vi "Select_Desired_Indicies.vi"(5 "No of averages":i32=1, 7 "Clients time":dbl, 8 "End time":dbl, 9 "Start time":dbl, 10 "Table values":dbl[][](array[numeric]) format="%.2f") -> (0 "Length":i32[](array[numeric]), 1 "End Integer":i32[](array[numeric]), 2 "Start integer":i32[](array[numeric]), 3 "Averaging Times":dbl[](array[numeric]) format="%.2f", 4 "Client leads me by:":dbl, 6 "Total Time":dbl format="%.2f")   [LabVIEW 2021]
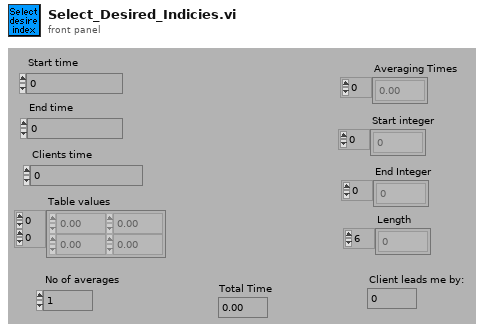
[diagram p1: front panel]
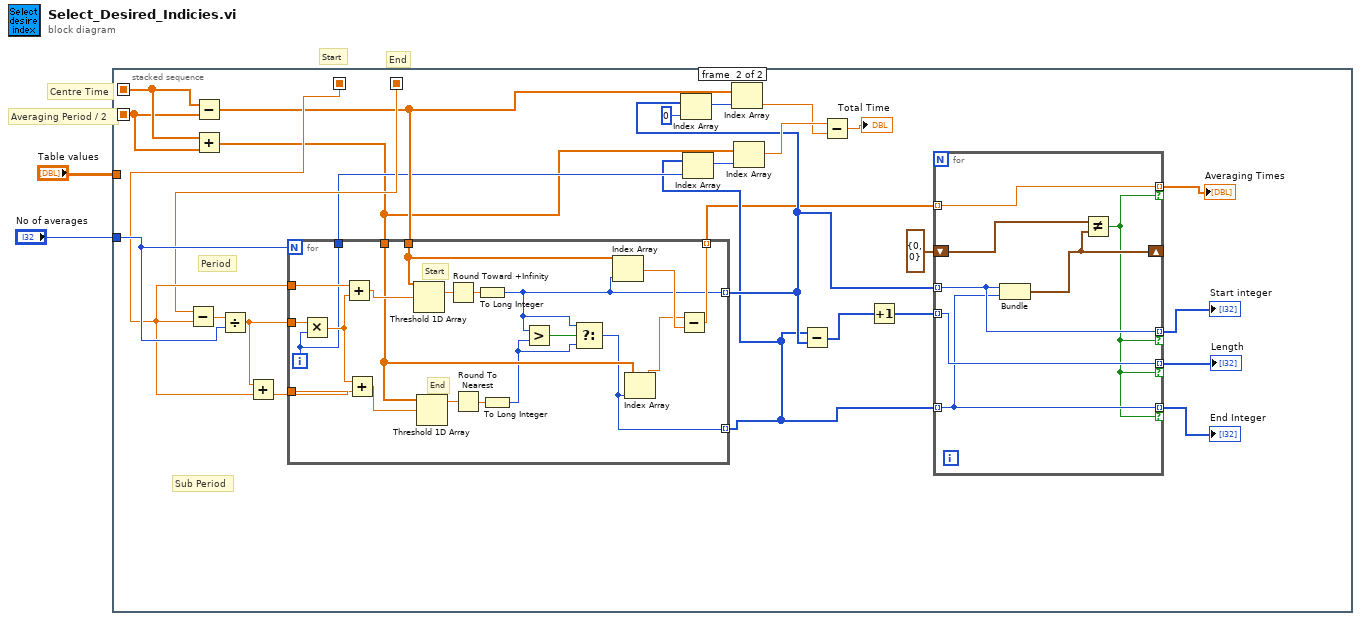
[diagram p0: block diagram]
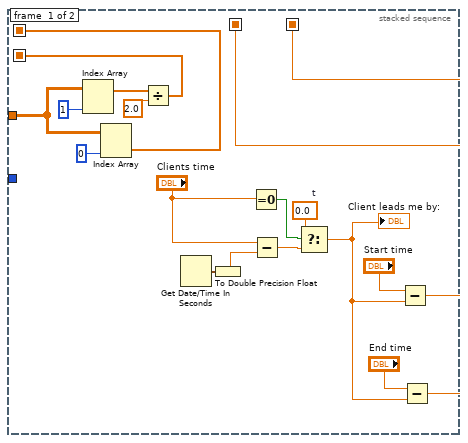
[diagram p2: hidden frame]
diagram:
  # "End"
  # "Start"
  # "Averaging Period / 2"
  # "Centre Time"
  n1 = stacked-sequence {
    seq-local: [w8 _] -> [_ w41]
    seq-local: [w12 _] -> [_ w43]
    seq-local: [w13 _] -> [_ w42]
    seq-local: [w4 _] -> [_ w40]
    tunnel: "Table values" -> [w9 _]
    tunnel: "No of averages" -> [_ w44]
    frame #0 {
      w14 = 0.0  # t
      n2 = Index Array(array=w9, index (col)=1) -> (element=w6:dbl[])  [unwired: 1 in]
      n3 = Index Array(array=w9, index (col)=0) -> (element=w8:dbl[])  [unwired: 1 in]
      n4 = Divide(x=w6, y=2.0) -> (x/y=w4:dbl[])
      n5 = Get Date/Time In Seconds() -> (seconds since 1Jan1904=w3:timestamp)
      n6 = To Double Precision Float(number=w3) -> (double precision float=w20:dbl)
      n7 = Equal To 0?(x="Clients time") -> (x = 0?=w15:bool)
      n8 = Subtract(x="Clients time", y=w20) -> (x-y=w16:dbl)
      n9 = Select(t=w14, s=w15, f=w16) -> (s? t:f=w7:dbl)
      "Client leads me by:" <- w7
      n10 = Subtract(x="Start time", y=w7) -> (x-y=w12:dbl)
      n11 = Subtract(x="End time", y=w7) -> (x-y=w13:dbl)
    }
    frame #1 {
      # "Sub Period"
      # "Period"
      n12 = Subtract(x=w42, y=w43) -> (x-y=w47:dbl)
      n13 = Subtract(x=w41, y=w40) -> (x-y=w37:dbl[])
      n14 = Add(x=w41, y=w40) -> (x+y=w34:dbl[])
      n15 = Divide(x=w47, y=w44) -> (x/y=w46:dbl)
      n16 = Add(x=w46, y=w43) -> (x+y=w45:dbl)
      n17 = for {
        N: w44 -> [_]
        tunnel: w46 -> [w74]
        tunnel: w43 -> [w73]
        tunnel: w45 -> [w71]
        tunnel: w37 -> [w65]
        tunnel: [w56] -> w26 mode=indexing
        tunnel: [w59] -> w25 mode=indexing
        tunnel: w34 -> [w66]
        tunnel: [w62] -> w22 mode=indexing
        tunnel: [w61] -> w35
        i -> [w61]
        # "End"
        # "Start"
        n18 = Multiply(x=w74, y=w61) -> (x*y=w72:dbl)
        n19 = Add(x=w73, y=w72) -> (x+y=w70:dbl)
        n20 = Add(x=w72, y=w71) -> (x+y=w67:dbl)
        n21 = Threshold 1D Array(2:w70, 3:w65) -> (0:w69:dbl)  [unwired: 1 out]
        n22 = Threshold 1D Array(2:w67, 3:w66) -> (0:w68:dbl)  [unwired: 1 out]
        n23 = Round Toward +Infinity(x=w69) -> (ceil(x): smallest int >= x=w58:dbl)
        n24 = Round To Nearest(number=w68) -> (nearest integer value=w57:dbl)
        n25 = To Long Integer(number=w58) -> (32bit integer=w56:i32)
        n26 = To Long Integer(number=w57) -> (32bit integer=w55:i32)
        n27 = Greater?(x=w56, y=w55) -> (0:w60:bool)
        n28 = Select(t=w56, s=w60, f=w55) -> (s? t:f=w59:i32)
        n29 = Index Array(array=w65, index=w56) -> (element=w64:dbl)
        n30 = Index Array(array=w66, index=w59) -> (element=w63:dbl)
        n31 = Subtract(x=w63, y=w64) -> (x-y=w62:dbl)
      }
      n32 = Index Array(array=w26, index=0 ("Index")) -> (element=w38:i32)
      n33 = Index Array(array=w25, index=w35) -> (element=w36:i32)
      n34 = Index Array(array=w37, index=w38) -> (element=w31:dbl)
      n35 = Index Array(array=w34, index=w36) -> (element=w32:dbl)
      n36 = Subtract(x=w25, y=w26) -> (x-y=w30:i32[])
      n37 = Subtract(x=w32, y=w31) -> (x-y=→"Total Time":dbl)
      n38 = Increment(x=w30) -> (x+1=w24:i32[])
      n39 = for {
        tunnel: w26 -> [w52] mode=indexing
        tunnel: w24 -> [w51] mode=indexing
        tunnel: w25 -> [w50] mode=indexing
        shift-right: [w54] -> _
        shift-left: cluster{i32, i32} {0, 0} -> [w53]
        tunnel: [w52] -> w27 mode=indexing if=w48
        tunnel: [w51] -> w28 mode=indexing if=w48
        tunnel: [w50] -> w29 mode=indexing if=w48
        tunnel: w22 -> [w49] mode=indexing
        tunnel: [w49] -> w21 mode=indexing if=w48
        n40 = Bundle(w52, w50) -> (w54:cluster{i32, i32})  [unwired: 1 in]
        n41 = Not Equal?(x=w53, y=w54) -> (x != y?=w48:bool)
      }
      "Averaging Times" <- w21
      "Start integer" <- w27
      "End Integer" <- w29
      "Length" <- w28
    }
  }
